vi "Hold.vi"(6 "Axis":T1, 8 "error in (no error)":errorcluster, 11 "Instrument.VRM in":refnum<class "Instrument.OxfordVRM.lvclass">) -> (0 "error out":errorcluster, 2 "Response":string, 3 "Instrument.VRM out":refnum<class "Instrument.OxfordVRM.lvclass">)   [LabVIEW 2019, in "Instrument.OxfordVRM.lvclass"]
uses:
  Instrument.OxfordVRM.lvclass
  Typedefs/VRM Magnet Axis--Enum.ctl
  <instrlib>/Mercury iXX/Public/Libraries/Magnet/Controls/PSU Actions.ctl
  Typedefs/Instrument.VRM.Commands-enum.ctl
  Typedefs/VRM Action-Axis--Cluster.ctl
  832d065b-a1a4-4964-bb06-cf8f55e9f82c.vi
  832d065b-a1a4-4964-bb06-cf8f55e9f82c.vi/28f5ceec-16db-4c68-850e-8a48c735b161.vi
  832d065b-a1a4-4964-bb06-cf8f55e9f82c.vi/28f5ceec-16db-4c68-850e-8a48c735b161.vi/91f4c535-94d6-4264-ad9c-e49c840c7187.vi
  832d065b-a1a4-4964-bb06-cf8f55e9f82c.vi/28f5ceec-16db-4c68-850e-8a48c735b161.vi/e39b395d-afff-419c-b8da-4829e0b8d408.vi
  832d065b-a1a4-4964-bb06-cf8f55e9f82c.vi/28f5ceec-16db-4c68-850e-8a48c735b161.vi/e39b395d-afff-419c-b8da-4829e0b8d408.vi/effd039b-3250-480c-8686-8c012769f095.vi
  <userlib>/LevyLab/Levylab Instruments/SMOs/RemoteControl/API/Remote Client.vi
  <vilib>/JDP Science/JSONtext/JSON text to Variant.vi
  <vilib>/JDP Science/JSONtext/LVClass Serializer/JSONtext LVClass Serializer.lvclass
  <instrlib>/Mercury iXX/Public/Libraries/Magnet.lvlib
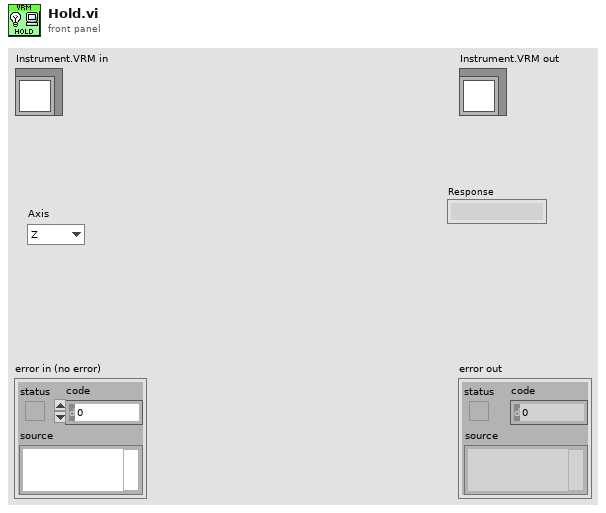
[diagram p1: front panel]
types:
  T1 = typedef "Instrument.OxfordVRM.lvclass/VRM Magnet Axis--Enum.ctl" = enum16{"Z", "X", "Y", "ALL"}
  T2 = typedef "Instrument.OxfordVRM.lvclass/VRM Action-Axis--Cluster.ctl" = cluster{"PSU Act Stat":T3, "Axis":T1}
  T3 = typedef "Mercury iXX.lvlib/Magnet.lvlib/PSU Actions.ctl" = string
  T4 = typedef "Instrument.OxfordVRM.lvclass/Instrument.VRM.Commands-enum.ctl" = enum16{"setAction", "setTarget", "setMagnetField", "getStatus", "getTarget", "getMagnetField"}
  T5 = cluster{"Holding":bool, "Ramp to Setpoint":bool, "Ramp to Zero":bool, "Clamp":bool}
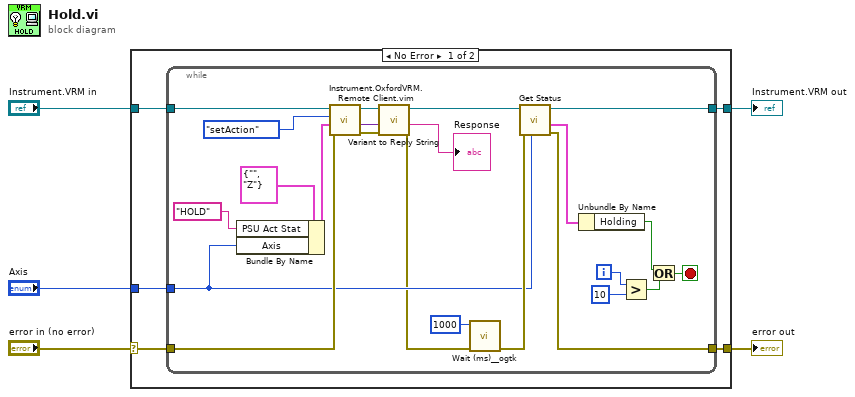
[diagram p0: block diagram]
diagram:
  n1 = case shown="No Error" "error in (no error)" {
    selector: "error in (no error)" -> [w9 w35]
    tunnel: [w7 w35] -> w4
    tunnel: [w8 w34] -> w2
    tunnel: "Instrument.VRM in" -> [w10 w34]
    tunnel: "Axis" -> [w6 _]
    frame No Error {
      n2 = while {
        tunnel: w6 -> [w13]
        tunnel: w10 -> [w28]
        tunnel: [w27] -> w8
        tunnel: w9 -> [w33]
        tunnel: [w32] -> w7
        i -> [w23]
        stop <- w24 stop-if-true
        n3 = Bundle By Name(cluster=T2 {"PSU Act Stat"="", "Axis"=enum."Z"}, "PSU Act Stat"=T3 "HOLD", "Axis"=w13) -> (w15:T2)
        n4 = call "Instrument.OxfordVRM.Remote Client.vim"("error in (no error)"=w33, "Data"=w15, "Commands"=Instrument.VRM.Commands-enum."setAction", "Instrument.VRM in"=w28) -> ("error out"=w18:errorcluster, "Data out"=w20:variant, "Instrument.VRM out"=w22:refnum<class "Instrument.OxfordVRM.lvclass">)  [unwired: 5 in]
        n5 = call "Variant to Reply String.vi"("error in (no error)"=w18, "Data"=w20, "Instrument.VRM in"=w22) -> ("error out"=w12:errorcluster, "Reply"=→"Response":string, "Instrument.VRM out"=w21:refnum<class "Instrument.OxfordVRM.lvclass">)  [unwired: 6 in]
        n6 = call <userlib>:"Wait (ms)__ogtk.vi"("error in (no error)"=w12, "milliseconds to wait"=u32 1000) -> ("error out"=w31:errorcluster)  [unwired: 8 in, 1 out]
        n7 = call "Get Status.vi"("Axis"=w13, "error in (no error)"=w31, "Instrument.VRM in"=w21) -> ("error out"=w32:errorcluster, "Status (ALL)"=w29:T5, "Instrument.VRM out"=w27:refnum<class "Instrument.OxfordVRM.lvclass">)  [unwired: 5 in, 1 out]
        n8 = Unbundle By Name(w29) -> ("Holding"=w11:bool)
        n9 = Greater?(x=w23, y=10) -> (0:w25:bool)
        n10 = Or(x=w11, y=w25) -> (x .or. y?=w24:bool)
      }
    }
    frame Error {
    }
  }
  "error out" <- w4
  "Instrument.VRM out" <- w2
